vi "optionsAcq_attenuatorAuto.vi"(8 "error in (no error)":errorcluster, 9 "readWrite":enum16{"read", "write"}(ring), 10 "auto":bool, 11 "Thorlabs_OSA_64 in":refnum<class "OSA.lvclass">) -> (0 "error out":errorcluster, 1 "status":string, 2 "auto out":bool, 3 "Thorlabs_OSA_64 out":refnum<class "OSA.lvclass">)   [LabVIEW 2010, in "OSA.lvclass"]
uses:
  OSA.lvclass
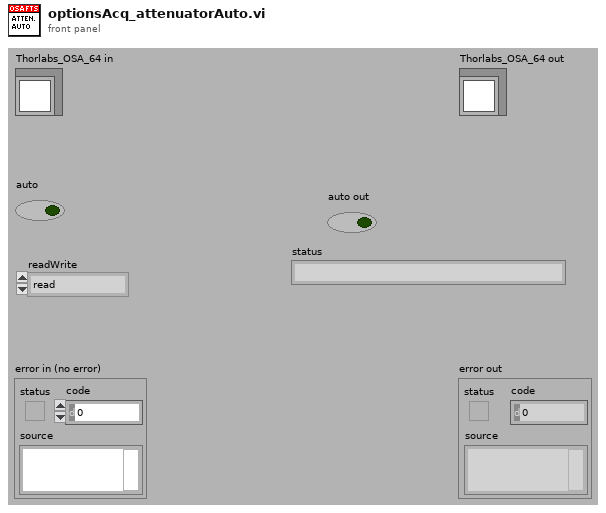
[diagram p1: front panel]
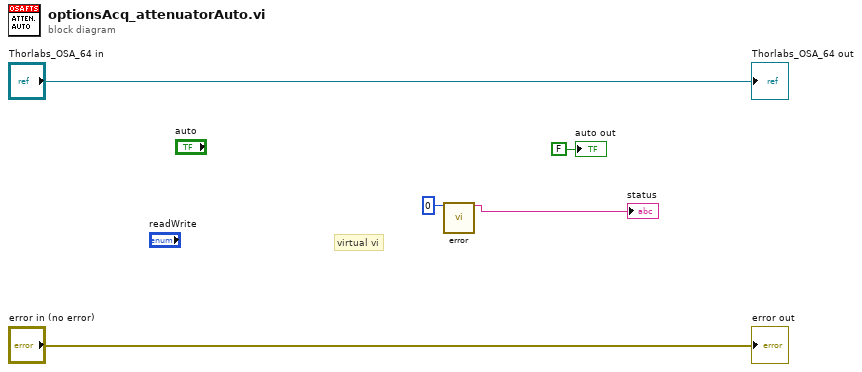
[diagram p0: block diagram]
diagram:
  # "virtual vi"
  n1 = call "error.vi"("result code"=0) -> ("status"=→"status":string)  [unwired: 16 in, 2 out]
  "error out" <- "error in (no error)"
  "Thorlabs_OSA_64 out" <- "Thorlabs_OSA_64 in"
  "auto out" <- FALSE ("auto out")
